vi "Desktop Main.vi"() -> ()   [LabVIEW 2018]
doc: "该模板是触摸面板模板的桌面部分。本模板基于队列消息处理器设计模式。\n\n事件处理循环负责按用户界面操作生成对应的消息。\n\n消息处理循环负责对事件处理循环或其他消息生成的消息进行处理。消息内容为字符串值，因此很容易将新消息添加至“消息处理”循环的“消息分支”条件结构。每个消息簇还能为消息数据提供可选值，该变体值可转换为要求的任何特定消息数据。\n\n通过共享变量对触摸面板终端的数据进行转换。"
uses:
  controls/UI Data.ctl
  support/Message Queue/Enqueue Message (Single).vi
  <vilib>/Utility/error.llb/Error Cluster From Error Code.vi
  <vilib>/ErrorRing/Error Ring.xnode
  support/Message Queue/Message Queue.lvlib
  support/User Event - Stop/User Event - Stop.lvlib
panel:
  out "数据":dbl(graph)
  in  "警告阈值<替换该项>":dbl=5.0 format="%#_13g"
  in  "退出":bool
  # "本模板基于队列消息处理器设计模式。\n\n关于该设计模式用法的更多信息，见队列消息处理器说明文档。"
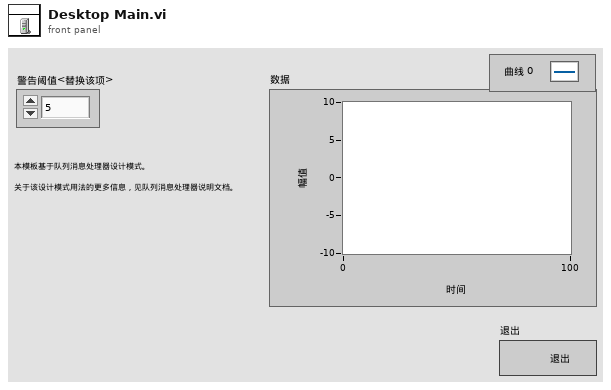
[diagram p1: front panel]
types:
  T1 = typedef "UI Data.ctl" = cluster{"警告阈值<替换该项>":refnum<vi>, "退出按钮引用":refnum<vi>}
  T2 = typedef "Message Queue.lvlib/All Message Queues.ctl" = cluster{"UI":refnum<queue>}
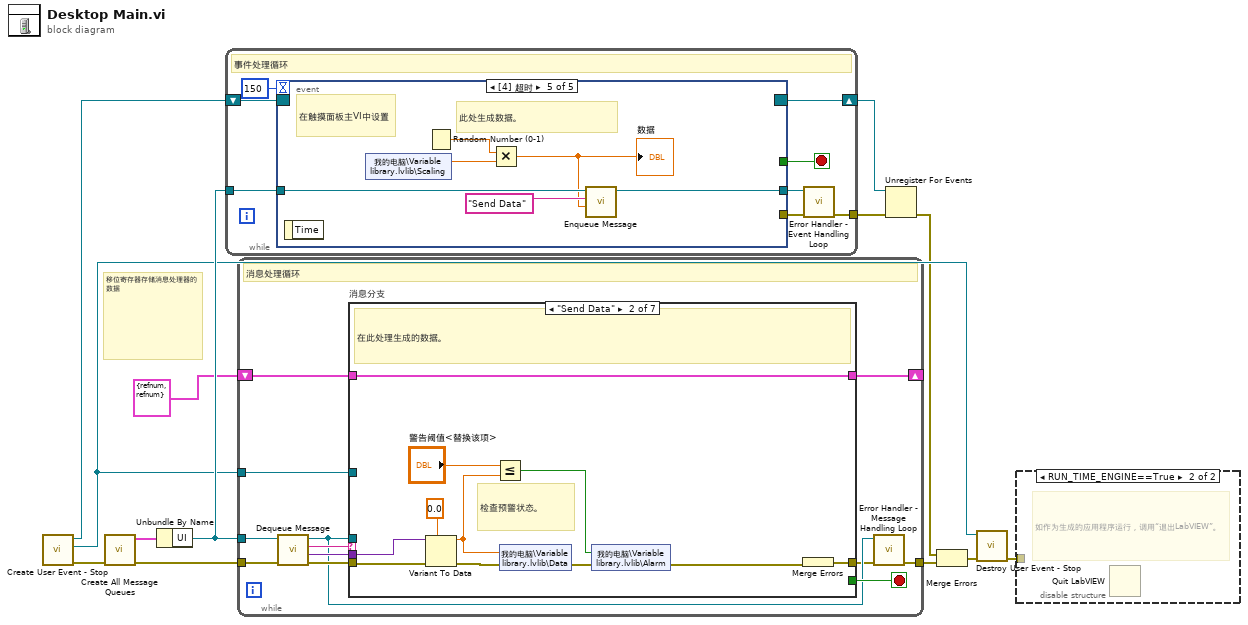
[diagram p0: block diagram]
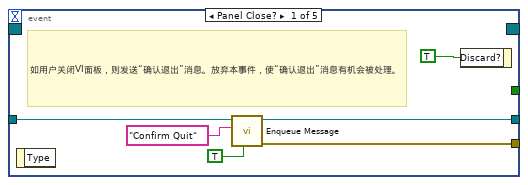
[diagram p3: hidden frame]
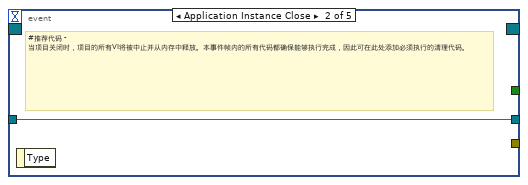
[diagram p4: hidden frame]
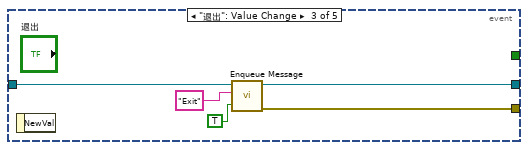
[diagram p5: hidden frame]
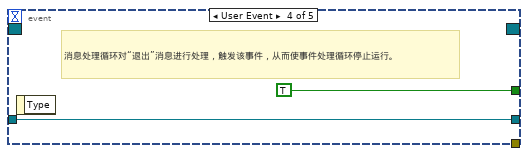
[diagram p6: hidden frame]
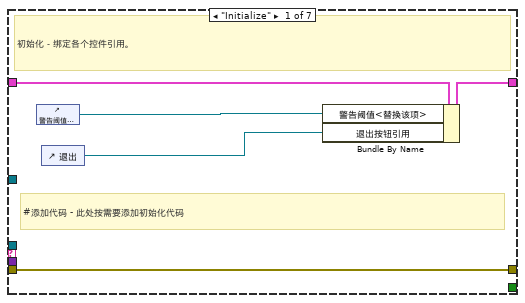
[diagram p7: hidden frame]
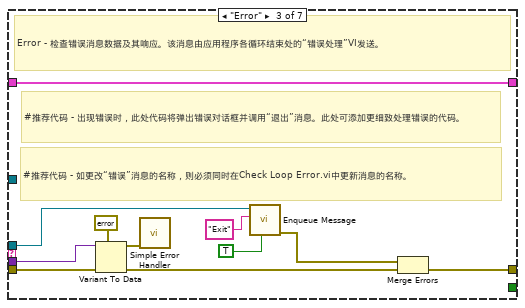
[diagram p8: hidden frame]
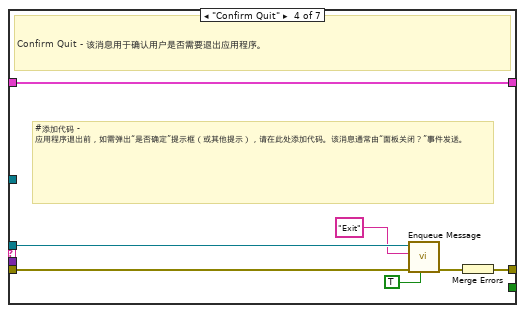
[diagram p9: hidden frame]
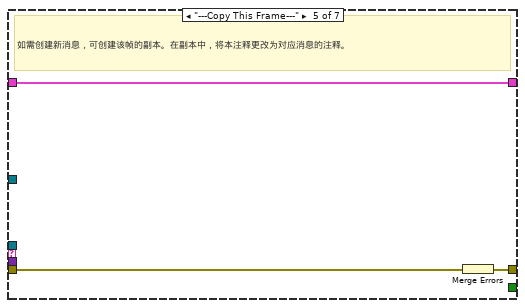
[diagram p10: hidden frame]
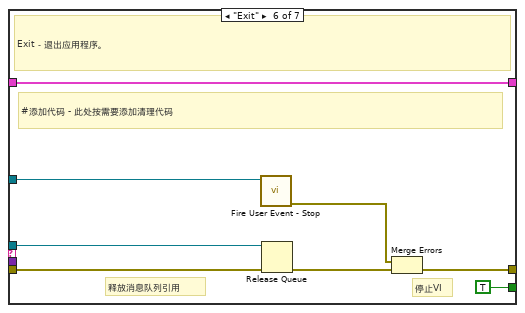
[diagram p11: hidden frame]
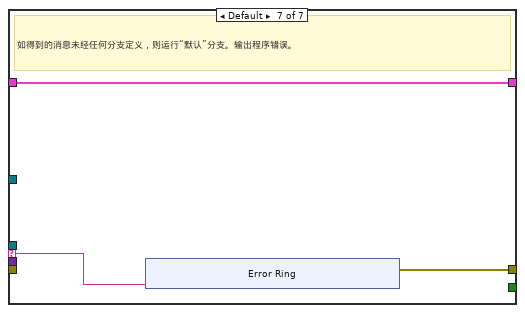
[diagram p12: hidden frame]
diagram:
  # "移位寄存器存储消息处理器的数据"
  n1 = call "Create User Event - Stop.vi"() -> ("error out"=w8:cluster{"状态":bool, "代码":i32, "源":string}, "用户事件－停止"=w6:refnum<user-event>, "停止事件注册引用句柄"=w9:refnum<event-registration>)  [unwired: 9 in]
  n2 = call "Create All Message Queues.vi"("error in (no error)"=w8) -> ("error out"=w13:cluster{"状态":bool, "代码":i32, "源":string}, "消息队列输出"=w12:T2)  [unwired: 9 in]
  n3 = Unbundle By Name(w12) -> ("UI"=w10:refnum<queue>)
  n4 = while {
    tunnel: w10 -> [w21]
    shift-right: [w19] -> w4
    shift-left: w9 -> [w20]
    tunnel: [w15] -> w1
    stop <- w17 stop-if-true
    # "事件处理循环"
    n5 = event shown="[4] 超时" {
      selector: w20 -> [_ _ _ _ _]
      dyn-events: [_ _ _ _ _] -> w19
      timeout: 150 -> [_ _ _ _ _]
      tunnel: [_ _ _ TRUE ("Discard?") _] -> w17
      tunnel: w21 -> [w26 w28 w33 w35 w41]
      tunnel: [w25 _ w32 _ _] -> w18
      tunnel: [w24 w28 w31 w35 w40] -> w16
      event Panel Close? {
        # "如用户关闭VI面板，则发送“确认退出”消息。放弃本事件，使“确认退出”消息有机会被处理。"
        n6 = event-data() -> ()  [unwired: 1 in, 1 out]
        n7 = call-poly "Enqueue Message.vi"("优先消息？ (F)"=TRUE ("Priority Message? (F)"), "消息"="Confirm Quit" ("Message"), "消息队列"=w26) -> ("error out"=w25:cluster{"状态":bool, "代码":i32, "源":string}, "消息队列副本"=w24:refnum<queue>)  [unwired: 7 in]
        n8 = event-data ("Event Filter Node")("Discard?"=TRUE) -> ()  [unwired: 1 in, 1 out]
      }
      event Application Instance Close {
        # "#推荐代码 - 当项目关闭时，项目的所有VI将被中止并从内存中释放。本事件帧内的所有代码都确保能够执行完成，因此可在此处添加必须执行的清理代码。"
        n9 = event-data() -> ()  [unwired: 1 in, 1 out]
      }
      event "退出": Value Change {
        n10 = event-data() -> ()  [unwired: 1 in, 1 out]
        n11 = call-poly "Enqueue Message.vi"("优先消息？ (F)"=TRUE ("Priority Message? (F)"), "消息"="Exit" ("Message"), "消息队列"=w33) -> ("error out"=w32:cluster{"状态":bool, "代码":i32, "源":string}, "消息队列副本"=w31:refnum<queue>)  [unwired: 7 in]
      }
      event User Event {
        # "消息处理循环对“退出”消息进行处理，触发该事件，从而使事件处理循环停止运行。"
        n12 = event-data() -> ()  [unwired: 1 in, 1 out]
      }
      event Timeout {
        # "在触摸面板主VI中设置"
        # "此处生成数据。"
        n13 = event-data() -> ()  [unwired: 1 in, 1 out]
        n14 = shared-variable "我的电脑\\Variable library.lvlib\\Scaling"() -> (w37:dbl)  [unwired: 1 in, 1 out]
        n15 = Random Number (0-1)() -> (number: 0 to 1=w38:dbl)
        n16 = Multiply(x=w38, y=w37) -> (x*y=w36:dbl)
        "数据" <- w36
        n17 = call-poly "Enqueue Message.vi"("消息数据"=w36, "消息"="Send Data" ("Message"), "消息队列"=w41) -> ("消息队列副本"=w40:refnum<queue>)  [unwired: 7 in, 1 out]
      }
    }
    n18 = call "Error Handler - Event Handling Loop.vi"("error in (no error)"=w18, "消息队列"=w16) -> ("错误输入副本"=w15:cluster{"状态":bool, "代码":i32, "源":string})  [unwired: 8 in, 1 out]
  }
  n19 = while {
    tunnel: w10 -> [w45]
    shift-right: [w52] -> _
    shift-left: T1 {"警告阈值<替换该项>"=refnum, "退出按钮引用"=refnum} ("Data Cluster") -> [w53]
    tunnel: w6 -> [w50]
    tunnel: w13 -> [w49]
    tunnel: [w43] -> w11
    stop <- w51 stop-if-true
    # "消息处理循环"
    n20 = call "Dequeue Message.vi"("error in (no error)"=w49, "消息队列"=w45) -> ("error out"=w48:cluster{"状态":bool, "代码":i32, "源":string}, "消息数据"=w46:variant, "消息"=w47:string, "消息队列副本"=w44:refnum<queue>)  [unwired: 6 in]
    n21 = case "消息分支" shown="\"Send Data\"" w47 {
      selector: w47 -> [_ _ _ _ _ _ w99]
      tunnel: w44 -> [_ _ w72 w83 _ w98 _]
      tunnel: w48 -> [w58 w65 w80 w87 w90 w93 _]
      tunnel: [w58 w68 w73 w85 w88 w94 w100] -> w42
      tunnel: w53 -> [w57 w69 w79 w86 w89 w97 w101]
      tunnel: [w56 w69 w79 w86 w89 w97 w101] -> w52
      tunnel: [_ _ _ _ _ TRUE _] -> w51
      tunnel: w46 -> [_ w63 w78 _ _ _ _]
      tunnel: w50 -> [_ _ _ _ _ w92 _]
      frame "Initialize" {
        # "#添加代码 - 此处按需要添加初始化代码"
        # "初始化－绑定各个控件引用。"
        n22 = control-ref of="警告阈值<替换该项>"() -> (w54:refnum<vi>)
        n23 = control-ref of="退出"() -> (w55:refnum<vi>)
        n24 = Bundle By Name(cluster=w57, "警告阈值<替换该项>"=w54, "退出按钮引用"=w55) -> (w56:T1)
      }
      frame "Send Data" {
        # "检查预警状态。"
        # "在此处理生成的数据。"
        n25 = Variant To Data(error in=w65, type=0.0 ("Data"), Variant=w63) -> (data=w61:dbl, error out=w60:errorcluster)
        n26 = Less Or Equal?(x="警告阈值<替换该项>", y=w61) -> (x <= y?=w66:bool)
        n27 = shared-variable "我的电脑\\Variable library.lvlib\\Data"(w61, error in=w60) -> (error out=w67:errorcluster)
        n28 = shared-variable "我的电脑\\Variable library.lvlib\\Alarm"(w66, error in=w67) -> (error out=w59:errorcluster)
        n29 = Merge Errors(w59) -> (w68:errorcluster)
      }
      frame "Error" {
        # "#推荐代码 - 如更改“错误”消息的名称，则必须同时在Check Loop Error.vi中更新消息的名称。"
        # "#推荐代码 - 出现错误时，此处代码将弹出错误对话框并调用“退出”消息。此处可添加更细致处理错误的代码。"
        # "Error - 检查错误消息数据及其响应。该消息由应用程序各循环结束处的“错误处理”VI发送。"
        n30 = Variant To Data(error in=w80, type=errorcluster {"status"=FALSE, "code"=0, "source"=""} ("error constant"), Variant=w78) -> (data=w76:errorcluster, error out=w75:errorcluster)
        n31 = call <vilib>:"Simple Error Handler.vi"("error in (no error)"=w76) -> ()  [unwired: 4 in, 5 out]
        n32 = call-poly "Enqueue Message.vi"("优先消息？ (F)"=TRUE ("Priority Message? (F)"), "消息"="Exit", "消息队列"=w72) -> ("error out"=w74:cluster{"状态":bool, "代码":i32, "源":string})  [unwired: 7 in, 1 out]
        n33 = Merge Errors(w74, w75) -> (w73:errorcluster)
      }
      frame "Confirm Quit" {
        # "#添加代码 - 应用程序退出前，如需弹出“是否确定”提示框（或其他提示），请在此处添加代码。该消息通常由“面板关闭？”事件发送。"
        # "Confirm Quit - 该消息用于确认用户是否需要退出应用程序。"
        n34 = call-poly "Enqueue Message.vi"("优先消息？ (F)"=TRUE ("Priority Message? (F)"), "error in (no error)"=w87, "消息"="Exit" ("Message"), "消息队列"=w83) -> ("error out"=w84:cluster{"状态":bool, "代码":i32, "源":string})  [unwired: 6 in, 1 out]
        n35 = Merge Errors(w84) -> (w85:errorcluster)
      }
      frame "---Copy This Frame---" {
        # "如需创建新消息，可创建该帧的副本。在副本中，将本注释更改为对应消息的注释。"
        n36 = Merge Errors(w90) -> (w88:errorcluster)
      }
      frame "Exit" {
        # "停止VI"
        # "释放消息队列引用"
        # "#添加代码 - 此处按需要添加清理代码"
        # "Exit－退出应用程序。"
        n37 = call "Fire User Event - Stop.vi"("用户事件－停止"=w92) -> ("error out"=w91:cluster{"状态":bool, "代码":i32, "源":string})  [unwired: 10 in]
        n38 = Release Queue(queue=w98, error in (no error)=w93) -> (error out=w95:errorcluster)  [unwired: 1 in, 2 out]
        n39 = Merge Errors(w91, w95) -> (w94:errorcluster)
      }
      frame Default {
        # "如得到的消息未经任何分支定义，则运行“默认”分支。输出程序错误。"
        n40 = xnode ("Error Ring")("参数 0"=w99) -> ("错误输出"=w100:errorcluster)
      }
    }
    n41 = call "Error Handler - Message Handling Loop.vi"("error in (no error)"=w42, "消息队列"=w44) -> ("错误输入副本"=w43:cluster{"状态":bool, "代码":i32, "源":string})  [unwired: 8 in, 1 out]
  }
  n42 = Unregister For Events(event registration refnum=w4, error in=w1) -> (error out=w5:errorcluster)
  n43 = Merge Errors(w5, w11) -> (w7:errorcluster)
  n44 = call "Destroy User Event - Stop.vi"("error in (no error)"=w7, "用户事件－停止"=w6) -> ("error out"=w2:cluster{"状态":bool, "代码":i32, "源":string})  [unwired: 9 in]
  n45 = disable-structure "Conditional Disable Structure" shown="RUN_TIME_ENGINE==True" {
    disable-tunnel: w2 -> [_ _]
    frame condition #0 (active) {
    }
    frame condition #1 {
      # "如作为生成的应用程序运行，调用“退出LabVIEW”。"
      n46 = Quit LabVIEW() -> ()  [unwired: 1 in]
    }
  }
